vi "VCS Set Current Must Ex.vi"(8 "error in (no error)":errorcluster, 10 "currentMust":i32, 11 "axis in":cluster{"keyHandle":u32, "nodeId":u16}={"keyHandle"=0, "nodeId"=1}) -> (0 "error out":errorcluster, 3 "axis out":cluster{"keyHandle":u32, "nodeId":u16}={"keyHandle"=0, "nodeId"=1})   [LabVIEW 2019, in "maxonEPOS.lvlib"]
doc: "<B>VCS Set Current Must</B> writes current mode demand value."
uses:
  Examples/maxonEPOS.lvlib
  Resources/EposCmd.dll
  Resources/EposCmd64.dll
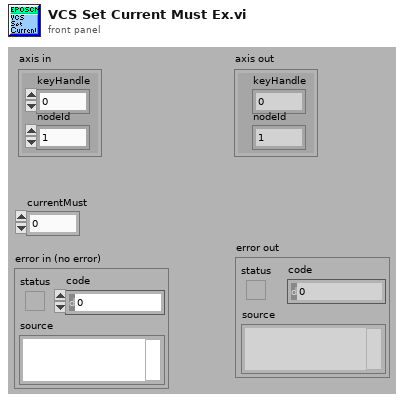
[diagram p1: front panel]
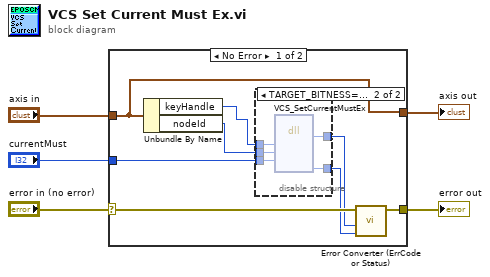
[diagram p0: block diagram]
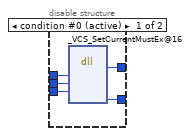
[diagram p2: hidden frame]
diagram:
  n1 = case shown="No Error" "error in (no error)" {
    selector: "error in (no error)" -> [w12 w25]
    tunnel: [w11 w25] -> w4
    tunnel: "currentMust" -> [w13 _]
    tunnel: "axis in" -> [w7 w24]
    tunnel: [w7 w24] -> w1
    frame No Error {
      n2 = Unbundle By Name(w7) -> ("keyHandle"=w9:u32, "nodeId"=w8:u16)
      n3 = disable-structure shown="TARGET_BITNESS==64" {
        disable-tunnel: w13 -> [w18 w23]
        disable-tunnel: [w17 w22] -> w10
        disable-tunnel: w9 -> [w16 w21]
        disable-tunnel: w8 -> [w15 w20]
        disable-tunnel: [w14 w19] -> w6
        frame condition #0 (active) {
          n4 = dll-call lib="C:/workspace/project/scancon/sw/SSI_Tool/InstrumentsInterfaces/Motordriver/maxon EPOS/Resources/EposCmd.dll" fn="_VCS_SetCurrentMustEx@16" ("EposCmd.dll:_VCS_SetVelocityMust@16")("KeyHandle"=w16, "NodeId"=w15, "CurrentMust"=w18) -> ("Rückgabetyp"=w14:i32, "pErrorCode"=w17:u32)  [unwired: 7 in, 2 out]
        }
        frame condition #1 {
          n5 = dll-call lib="C:/Sources/LabView/maxon EPOS/Resources/EposCmd64.dll" fn="VCS_SetCurrentMustEx" ("EposCmd.dll:_VCS_SetVelocityMust@16")("KeyHandle"=w21, "NodeId"=w20, "CurrentMust"=w23) -> ("Rückgabetyp"=w19:i32, "pErrorCode"=w22:u32)  [unwired: 7 in, 2 out]
        }
      }
      n6 = call "Error Converter (ErrCode or Status).vi"("error code"=w10, "return type"=w6, "error in (no error)"=w12) -> ("error out"=w11:errorcluster)  [unwired: 7 in]
    }
    frame Error {
    }
  }
  "error out" <- w4
  "axis out" <- w1
